vi "Disabled.vi"(7 "Robot Mode":T3, 10 "Match Info":T2={"Autonomous Elapsed Seconds"=0.0, "TeleOp Elapsed Seconds"=0.0, "Disabled Elapsed Seconds"=0.0, "Visited Autonomous"=FALSE, "Visited TeleOp"=FALSE, "Visited Disabled"=FALSE, "Autonomous Settings"={"Autonomous Style"=enum."Independent", "VI Refnum"=refnum}}, 11 "Call Context":T4) -> ()   [LabVIEW 2011]
doc: "This VI is called each time a disabled packet is received from the DS. It is often used to prepare for the next robot mode, to calibrate sensors, etc."
uses:
  <vilib>/Rock Robotics/WPI/DriverStation/WPI_DriverStationDerivedRobotMode.ctl
  <vilib>/Rock Robotics/WPI/DriverStation/WPI_DriverStationRobotMode.ctl
  <vilib>/Rock Robotics/WPI/DriverStation/WPI_DriverStationMatch Info.ctl
  <vilib>/Rock Robotics/WPI/Joystick/WPI_JoystickButtonState.ctl
  Robot Global Data.vi
panel:
  out "Buttons 2":T1
  out "Buttons":T1
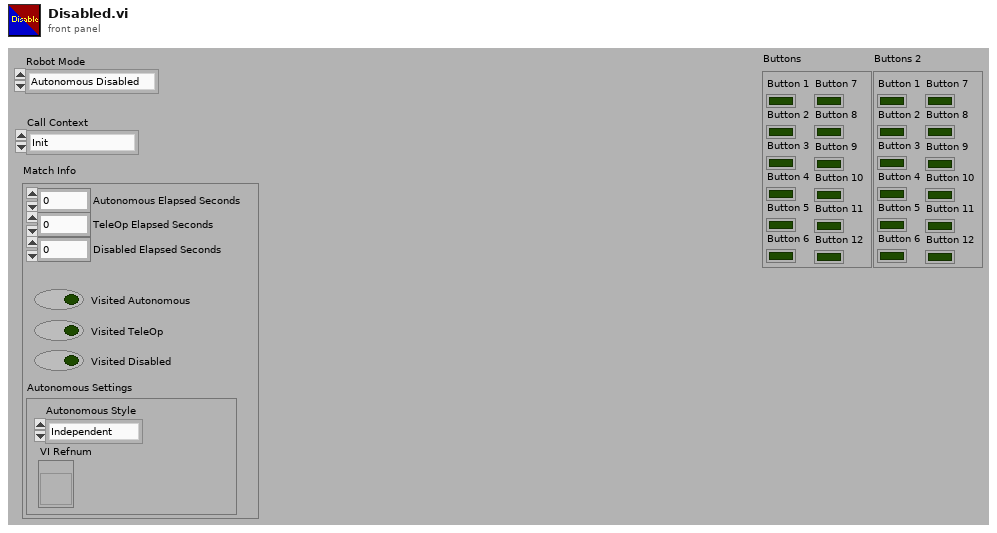
[diagram p1: front panel]
types:
  T1 = typedef "WPI_JoystickButtonState.ctl" = cluster{"Button 1":bool, "Button 2":bool, "Button 3":bool, "Button 4":bool, "Button 5":bool, "Button 6":bool, "Button 7":bool, "Button 8":bool, "Button 9":bool, "Button 10":bool, "Button 11":bool, "Button 12":bool}
  T2 = typedef "WPI_DriverStationMatch Info.ctl" = cluster{"Autonomous Elapsed Seconds":dbl, "TeleOp Elapsed Seconds":dbl, "Disabled Elapsed Seconds":dbl, "Visited Autonomous":bool, "Visited TeleOp":bool, "Visited Disabled":bool, "Autonomous Settings":cluster{"Autonomous Style":enum16{"Iterative", "Independent"}, "VI Refnum":refnum<vi>}}
  T3 = typedef "WPI_DriverStationRobotMode.ctl" = enum16{"Autonomous Disabled", "Autonomous Enabled", "Teleop Disabled", "Teleop Enabled", "Timeout", "Finish"}
  T4 = typedef "WPI_DriverStationDerivedRobotMode.ctl" = enum16{"Init", "Execute", "Stop"}
  T5 = typedef "WPI_JoystickDevRef.ctl" = cluster{"Device":T6}
  T6 = typedef "WPI_JoystickDeviceEnum.ctl" = enum16{"USB 1", "USB 2", "USB 3", "USB 4", "Kinect 1", "Kinect 2"}
  T7 = typedef "WPI_EncoderDevRef.ctl" = cluster{"DevStatus":errorcluster, "EncoderIndex":T8, "CounterIndex":T9, "DistancePerCount":dbl, "Decoding Type":T10}
  T8 = typedef "FPGA_EncoderIdx.ctl" = enum8{"Enc 0", "Enc 1", "Enc 2", "Enc 3", "Invalid"}
  T9 = typedef "FPGA_CounterCtrSystemIndex.ctl" = enum8{"Ctr 0", "Ctr 1", "Ctr 2", "Ctr 3", "Ctr 4", "Ctr 5", "Ctr 6", "Ctr 7", "Invalid"}
  T10 = typedef "WPI_EncoderType.ctl" = enum16{"1x", "2x", "4x"}
  T11 = typedef "WPI_GyroDevRef.ctl" = cluster{"DevStatus":errorcluster, "Analog Module":T12, "Analog Channel":T13, "Offset":dbl, "Gain (VoltsPerDegree/Second)":dbl}
  T12 = typedef "FPGA_TypedefAnalogModule.ctl" = enum16{"Analog Module 1", "Analog Module 2"}
  T13 = typedef "FPGA_AIChannel.ctl" = enum8{"AI 1", "AI 2", "AI 3", "AI 4", "AI 5", "AI 6", "AI 7", "AI 8", "Invalid"}
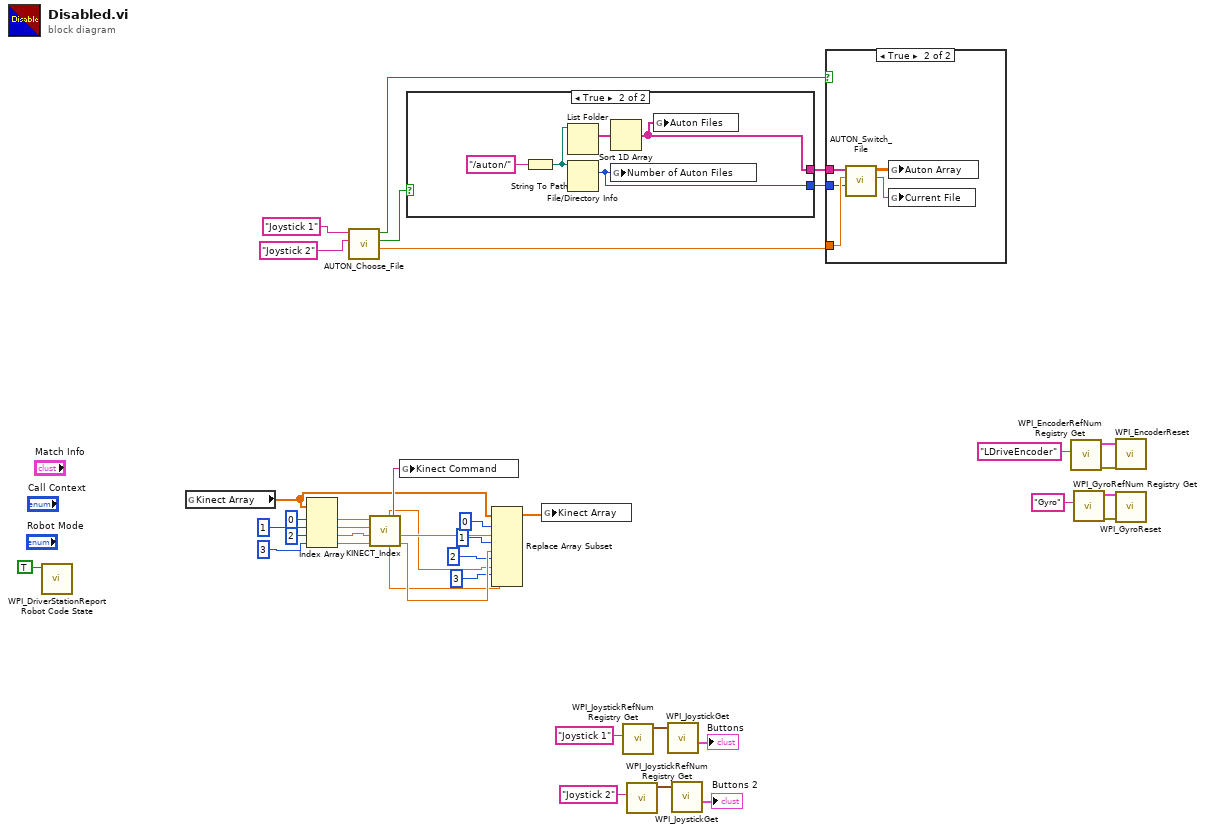
[diagram p0: block diagram]
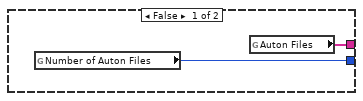
[diagram p3: hidden frame]
diagram:
  n1 = call <vilib>:"WPI_DriverStationReport Robot Code State.vi"("Disabled"=TRUE ("Autonomous")) -> ()  [unwired: 10 in, 1 out]
  n2 = global read "Robot Global Data.vi" "Kinect Array"() -> (w29:dbl[])
  n3 = Index Array(array=w29, index #1=0 ("index"), index #2=1 ("index"), index #3=2 ("index"), index #4=3 ("index")) -> (element #1=w33:dbl, element #2=w32:dbl, element #3=w31:dbl, element #4=w30:dbl)
  n4 = call "AUTON_Choose_File.vi"("Joystick 2 Refnum"="Joystick 2" ("refnum name"), "Joystick 1 Refnum"="Joystick 1" ("refnum name")) -> ("Auton File"=w1:dbl, "Refresh"=w3:bool, "Allow Change"=w2:bool)  [unwired: 7 in]
  n5 = call "KINECT_Index.vi"("Arm Drive Min in (Reverse)"=w30, "Arm Drive Max in (Forward)"=w31, "Z Wrist Left"=w32, "Z Wrist Right"=w33) -> ("Z Wrist Left"=w25:sgl, "Z Wrist Right"=w27:sgl, "Kinect Command"=w38:string, "Arm Drive Min out (Reverse)"=w21:dbl, "Arm Drive Max out (Forward)"=w22:dbl)  [unwired: 3 in]
  n6 = global write "Robot Global Data.vi" "Kinect Command"(w38) -> ()
  n7 = case shown="True" w3 {
    tunnel: [w40 w43] -> w12
    tunnel: [w41 w42] -> w13
    frame False {
      n8 = global read "Robot Global Data.vi" "Number of Auton Files"() -> (w40:i64)
      n9 = global read "Robot Global Data.vi" "Auton Files"() -> (w41:string[])
    }
    frame True {
      n10 = String To Path(string="/auton/") -> (path=w45:path)
      n11 = List Folder(path=w45) -> (filenames=w44:string[])  [unwired: 1 in, 5 out]
      n12 = File/Directory Info(path=w45) -> (size=w43:i64)  [unwired: 1 in, 6 out]
      n13 = Sort 1D Array(array=w44) -> (sorted array=w42:string[])
      n14 = global write "Robot Global Data.vi" "Number of Auton Files"(w43) -> ()
      n15 = global write "Robot Global Data.vi" "Auton Files"(w42) -> ()
    }
  }
  n16 = Replace Array Subset(array=w29, new element #1=w27, index #1=0 ("index"), new element #2=w25, index #2=1 ("index"), new element #3=w22, index #3=2 ("index"), new element #4=w21, index #4=3 ("index")) -> (w20:dbl[])
  n17 = global write "Robot Global Data.vi" "Kinect Array"(w20) -> ()
  n18 = call <vilib>:"WPI_JoystickRefNum Registry Get.vi"("refnum name"="Joystick 1") -> ("JoystickDevRef"=w19:T5)  [unwired: 9 in, 1 out]
  n19 = call <vilib>:"WPI_JoystickRefNum Registry Get.vi"("refnum name"="Joystick 2") -> ("JoystickDevRef"=w16:T5)  [unwired: 9 in, 1 out]
  n20 = call <vilib>:"WPI_JoystickGet.vi"("JoystickDevRef"=w19) -> ("Buttons"=→"Buttons":T1)  [unwired: 4 in, 2 out]
  n21 = call <vilib>:"WPI_JoystickGet.vi"("JoystickDevRef"=w16) -> ("Buttons"=→"Buttons 2":T1)  [unwired: 4 in, 2 out]
  n22 = case shown="True" w2 {
    tunnel: w1 -> [_ w49]
    tunnel: w13 -> [_ w48]
    tunnel: w12 -> [_ w47]
    frame False {
    }
    frame True {
      n23 = call "AUTON_Switch_File.vi"("Number of Auton Files"=w47, "Auton File"=w49, "Auton Files"=w48) -> ("Current File"=w50:string, "Auton Array"=w51:dbl[][])  [unwired: 7 in]
      n24 = global write "Robot Global Data.vi" "Auton Array"(w51) -> ()
      n25 = global write "Robot Global Data.vi" "Current File"(w50) -> ()
    }
  }
  n26 = call <vilib>:"WPI_EncoderRefNum Registry Get.vi"("refnum name"="LDriveEncoder") -> ("error out"=w11:errorcluster, "EncoderDevRef"=w10:T7)  [unwired: 9 in]
  n27 = call <vilib>:"WPI_GyroRefNum Registry Get.vi"("refnum name"="Gyro") -> ("error out"=w8:errorcluster, "GyroDevRef"=w9:T11)  [unwired: 9 in]
  n28 = call <vilib>:"WPI_EncoderReset.vi"("error in (no error)"=w11, "EncoderDevRef"=w10) -> ()  [unwired: 8 in, 2 out]
  n29 = call <vilib>:"WPI_GyroReset.vi"("error in (no error)"=w8, "GyroDevRef"=w9) -> ()  [unwired: 8 in, 2 out]
